vi "Normalize.vi"(2 "A":T1={"Array Num"=[1, 2, 3], "Decimal Index"=0, "stop"=FALSE}) -> (0 "Normalized A":T1={"Array Num"=[1, 2, 3], "Decimal Index"=0, "stop"=FALSE})   [LabVIEW 2025]
uses:
  Number.ctl
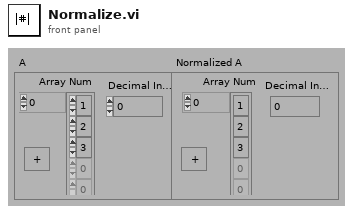
[diagram p1: front panel]
types:
  T1 = typedef "Number.ctl" = cluster{"Array Num":i8[], "Decimal Index":i32, "stop":bool}
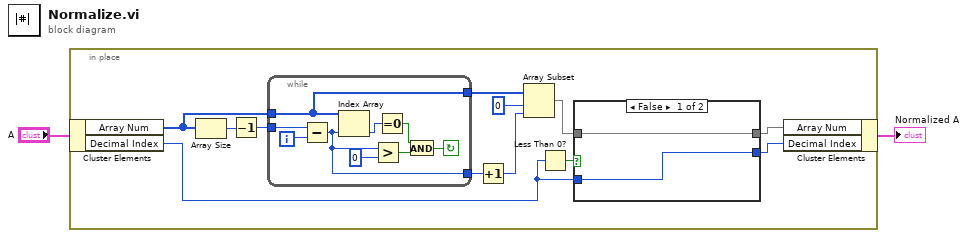
[diagram p0: block diagram]
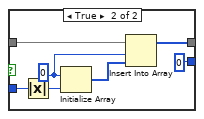
[diagram p2: hidden frame]
diagram:
  n1 = in-place {
    n2 = in-place-cluster #1("A") -> ("Array Num"=w6:i8[], "Decimal Index"=w5:i32)
    n3 = Array Size(array=w6) -> (size(s)=w12:i32)
    n4 = Decrement(x=w12) -> (x-1=w13:i32)
    n5 = while {
      tunnel: [w21] -> w11
      tunnel: [w16] -> w10
      tunnel: w13 -> [w23]
      tunnel: w6 -> [w21]
      i -> [w20]
      stop <- w17 continue-if-true
      n6 = Subtract(x=w23, y=w20) -> (x-y=w16:i32)
      n7 = Index Array(array=w21, index=w16) -> (element=w22:i8)
      n8 = Greater?(x=w16, y=0) -> (0:w19:bool)
      n9 = Equal To 0?(x=w22) -> (x = 0?=w18:bool)
      n10 = And(x=w18, y=w19) -> (x .and. y?=w17:bool)
    }
    n11 = Increment(x=w10) -> (x+1=w8:i32)
    n12 = Array Subset(array=w11, index=0, length=w8) -> (w9:i8[])
    n13 = Less Than 0?(x=w5) -> (x < 0?=w14:bool)
    n14 = case shown="False" w14 {
      tunnel: w9 -> [w25 w28]
      tunnel: w5 -> [w24 w31]
      tunnel: [w25 w29] -> w4
      tunnel: [w24 i8 0] -> w3
      frame False {
      }
      frame True {
        w26 = i8 0
        n15 = Absolute Value(x=w31) -> (abs(x)=w32:i32)
        n16 = Initialize Array(w26, w32) -> (w27:i8[])
        n17 = Insert Into Array(array=w28, index=w26, new element=w27) -> (w29:i8[])
      }
    }
    n18 = in-place-cluster #1("Array Num"=w4, "Decimal Index"=w3) -> (→"Normalized A":T1)
  }
